vi "Auto_Routine_DepositBalance.vi"(8 "error in (no error)":errorcluster) -> (0 "error out":errorcluster)   [LabVIEW 2020]
doc: "Deposites a cone on the upper node then balances\nInputs:\n--ErrorIn--\nOutputs:\n--ErrorOut--"
uses:
  Arm/ArmPositionPreset.ctl
  Arm/ArmGamePiecePreset.ctl
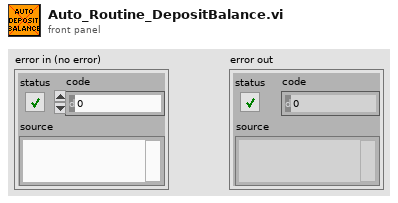
[diagram p1: front panel]
types:
  T1 = typedef "ArmGamePiecePreset.ctl" = enum16{"Cube", "Cone"}
  T2 = typedef "ArmPositionPreset.ctl" = enum16{"Upper", "Lower", "Middle", "Home", "Shelf", "Floor", "HalfFloor", "HalfHome"}
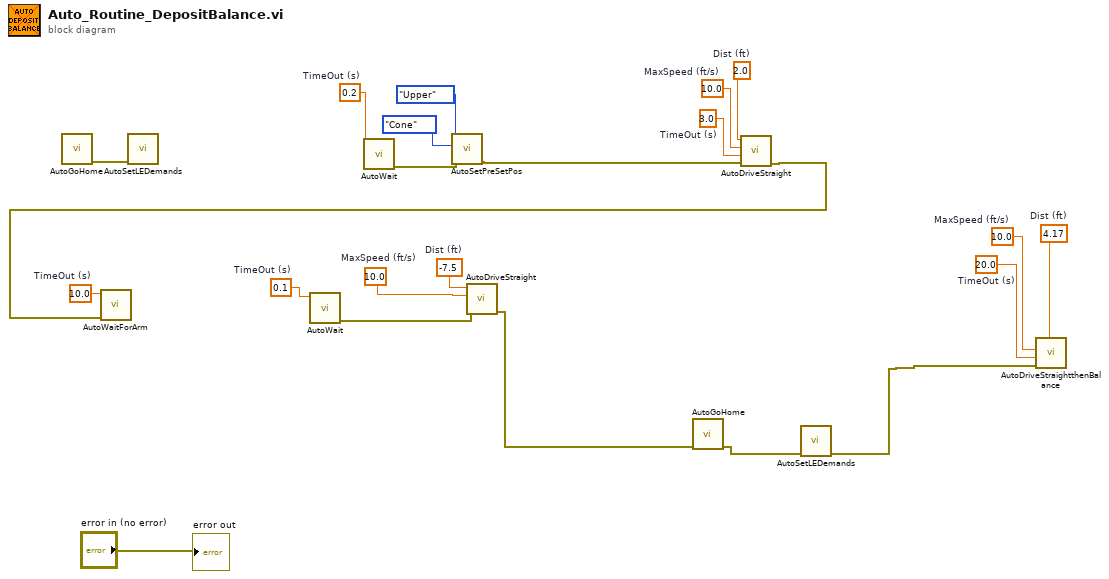
[diagram p0: block diagram]
diagram:
  w18 = 20.0  # TimeOut (s)
  w17 = 4.17  # Dist (ft)
  w16 = 10.0  # MaxSpeed (ft/s)
  w15 = 10.0  # MaxSpeed (ft/s)
  w22 = 3.0  # TimeOut (s)
  w21 = 10.0  # MaxSpeed (ft/s)
  w20 = 2.0  # Dist (ft)
  w13 = -7.5  # Dist (ft)
  w12 = 0.1  # TimeOut (s)
  w11 = 10.0  # TimeOut (s)
  w9 = 0.2  # TimeOut (s)
  n1 = call "AutoGoHome.vi"() -> ("error out"=w1:errorcluster)  [unwired: 11 in]
  n2 = call "AutoSetLEDemands.vi"("error in (no error)"=w1) -> ()  [unwired: 10 in, 1 out]
  n3 = call "AutoWait.vi"("TimeOut (s)"=w12) -> ("error out"=w14:errorcluster)  [unwired: 10 in]
  n4 = call "AutoWait.vi"("TimeOut (s)"=w9) -> ("error out"=w10:errorcluster)  [unwired: 10 in]
  n5 = call "AutoSetPreSetPos.vi"("error in (no error)"=w10, "Game Piece"=ArmGamePiecePreset."Cone", "Position"=ArmPositionPreset."Upper") -> ("error out"=w4:errorcluster)  [unwired: 8 in]
  n6 = call "AutoDriveStraight.vi"("error in (no error)"=w14, "MaxSpeed (ft/s)"=w15, "Dist (ft)"=w13) -> ("error out"=w2:errorcluster)  [unwired: 8 in]
  n7 = call "AutoGoHome.vi"("error in (no error)"=w2) -> ("error out"=w3:errorcluster)  [unwired: 10 in]
  n8 = call "AutoDriveStraight.vi"("error in (no error)"=w4, "TimeOut (s)"=w22, "MaxSpeed (ft/s)"=w21, "Dist (ft)"=w20) -> ("error out"=w19:errorcluster)  [unwired: 7 in]
  n9 = call "AutoWaitForArm.vi"("error in (no error)"=w19, "TimeOut (s)"=w11) -> ()  [unwired: 9 in, 1 out]
  n10 = call "AutoSetLEDemands.vi"("error in (no error)"=w3) -> ("error out"=w5:errorcluster)  [unwired: 10 in]
  n11 = call "AutoDriveStraightthenBalance.vi"("error in (no error)"=w5, "TimeOut (s)"=w18, "MaxSpeed (ft/s)"=w16, "Dist (ft)"=w17) -> ()  [unwired: 7 in, 1 out]
  "error out" <- "error in (no error)"
